vi "measurementGlobal.vi"() -> ()   [LabVIEW 2013]
panel:
  in  "Tab Control":enum32{"General", "DAQ"}(tab)
  in  "Current No of Blocks":i32
  in  "Input No of Blocks":i32
  in  "Input No of samples":i32
  in  "Input Sampling rate (Hz)":dbl
  in  "Actual Measurement time (mins)":dbl
  in  "Average time (mins)":dbl
  in  "?":i16(ring) items=["Acquire Data"]
  in  "Task Name":string
  out "Chan + Span Limit":T1(array[cluster])
  in  "Analogue Data (volts)":dbl[][](array[numeric])
  out "taskReadInputs":refnum<k21>
  in  "sample mode":i32(ring)=10178 items=["Finite Samples"=10178, "Continuous Samples"=10123, "Hardware Timed Single Point"=12522]
  in  "input terminal configuration":i32(ring)=-1 items=["Default"=-1, "RSE"=10083, "NRSE"=10078, "Differential"=10106, "Pseudodifferential"=12529]
  in  "NI Device Name":string
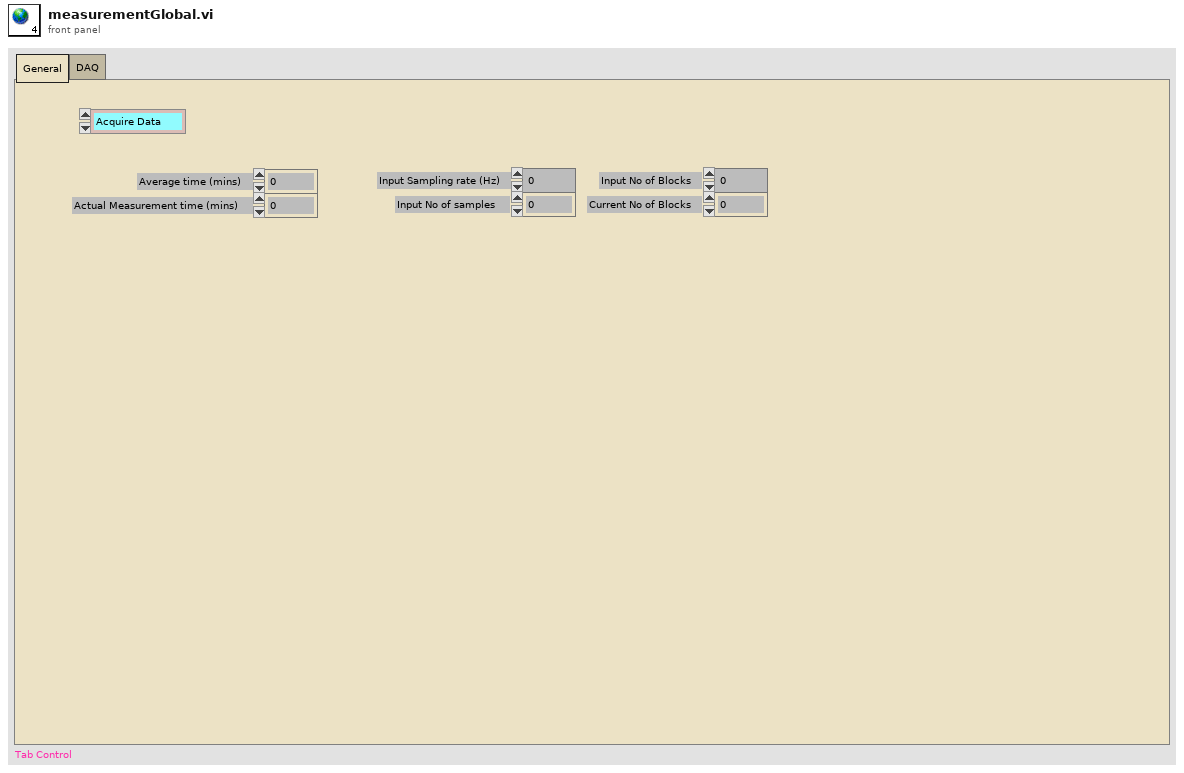
[diagram p1: front panel]
types:
  T1 = cluster{"Chan No":i32, "Low Volt Limit (-10V)":dbl, "High Volt Limit (10V)":dbl}[]
diagram:
